vi "apply key value pairs.vi"(8 "error in":errorcluster, 9 "values":string[](array[string]), 10 "keys":string[](array[string]), 11 "fixed channel runtime in":refnum<class "control module runtime.lvclass">) -> (0 "error out":errorcluster, 3 "fixed channel runtime out":refnum<class "control module runtime.lvclass">)   [LabVIEW 2013, in "control module runtime.lvclass"]
uses:
  control module runtime.lvclass
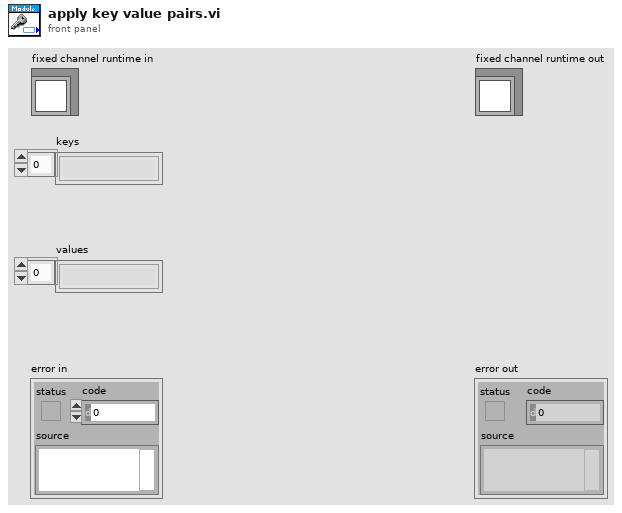
[diagram p1: front panel]
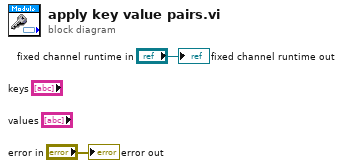
[diagram p0: block diagram]
diagram:
  "error out" <- "error in"
  "fixed channel runtime out" <- "fixed channel runtime in"
